vi "Read&Write.vi"(6 "In":u8=130 format="%.0x", 8 "error in (no error)":errorcluster={"status"=TRUE, "code"=56, "source"="UDP Read in UDP.vi->Read&Write.vi->Untitled 1"}, 9 "Address":u32=2305 format="%x", 10 "Read (TRUE)":bool, 11 "address":string="192.168.10.35") -> (0 "error out":errorcluster={"status"=TRUE, "code"=56, "source"="UDP Read in UDP.vi->Read&Write.vi->Untitled 1"}, 2 "Out":u8 format="%.0x")   [LabVIEW 2017]
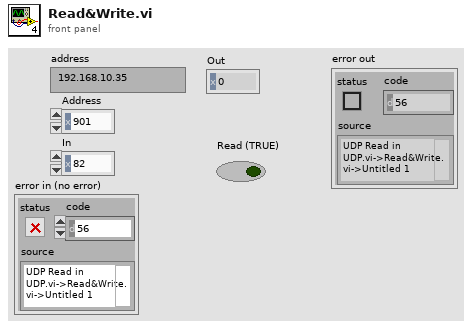
[diagram p1: front panel]
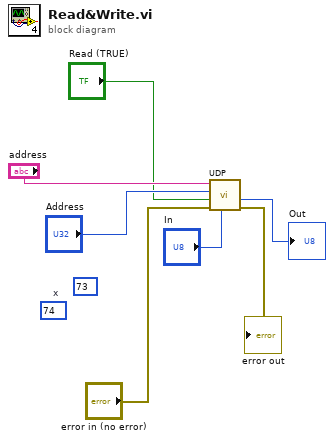
[diagram p0: block diagram]
diagram:
  (unwired) u32 73 ("Address")
  (unwired) u16 74  # x
  n1 = call "UDP.vi"("In"="In", "error in (no error)"="error in (no error)", "Read (TRUE)"="Read (TRUE)", "Address"="Address", "IP address"="address") -> ("error out"=→"error out":errorcluster, "Out"=→"Out":u8)  [unwired: 3 in, 1 out]
